vi "DetermineCurrentRegime.vi"(10 "Robot Heading (deg)":dbl, 11 "Trusted Absolute Wind Data (deg)":dbl) -> (3 "Sailing Regime":T1)   [LabVIEW 2013]
doc: "This VI looks at the robot state (heading and wind) and determines which boat regime we are currently in, ignoring whether or not we are in a transition. It ignores the transistions because another section of the code checks whether we are in a transition and does that based on that last commanded regime, not based on the current absolute wind vs. heading of the robot.\n\nEric Schneider, Feb. 2014"
uses:
  Data/TypeDefs/Sailing Regimes.ctl
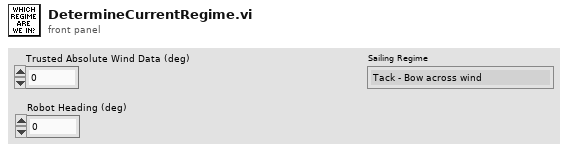
[diagram p1: front panel]
types:
  T1 = typedef "Sailing Regimes.ctl" = enum16{"Tack - Bow across wind", "Upwind - Port Tack", "Turn between Upwind/Reach - Port Tack", "Reach - Port Tack", "Turn between Reach/Run - Port Tack", "Run - Port Tack", "Jibe - Stern across wind", "Run - Starboard Tack", "Turn between Reach/Run - Starboard Tack", "Reach - Starboard Tack", "Turn between Upwind/Reach - Starboard Tack", "Upwind - Starboard Tack"}
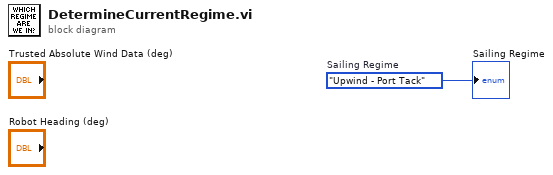
[diagram p0: block diagram]
diagram:
  w1 = Sailing_Regimes."Upwind - Port Tack"  # Sailing Regime
  "Sailing Regime" <- w1
